vi "CreateCANWriteQueues.vi"(8 "error in (no error)":errorcluster, 10 "CAN frame":T1 {"type" items=["CAN Data", "CAN Remote"]; "identifier" format="%.0x"}, 11 "Queues":refnum<queue>) -> (0 "error out":errorcluster, 3 "Queues":refnum<queue>)   [LabVIEW 2016, in "DSI-RT.lvlib"]
uses:
  DSI-RT.lvlib
  <vilib>/RioEmbeddedCAN/RioEmbeddedCAN.llb/CANFrameControl.ctl
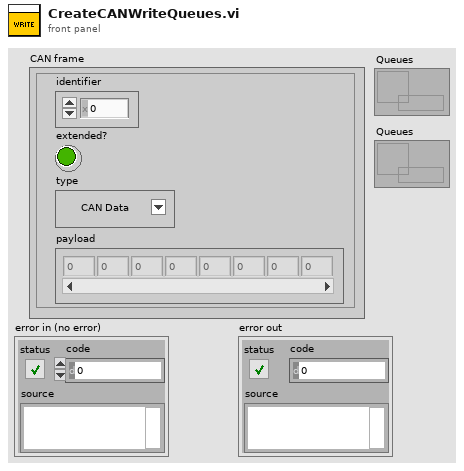
[diagram p1: front panel]
types:
  T1 = typedef "CANFrameControl.ctl" = cluster{"identifier":u32, "extended?":bool, "type":u8, "payload":u8[]}
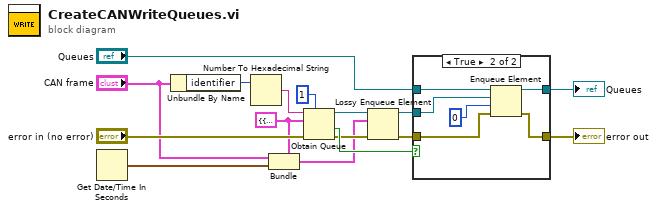
[diagram p0: block diagram]
diagram:
  w3 = cluster{"CAN frame":T1, "Timestamp":timestamp} {"CAN frame"={"identifier"=0, "extended?"=FALSE, "type"=0, "payload"=[]}, "Timestamp"=timestamp(0 s since 1904-01-01)} ("output cluster")
  n1 = Get Date/Time In Seconds() -> (seconds since 1Jan1904=w14:timestamp)
  n2 = Unbundle By Name("CAN frame") -> ("identifier"=w12:u32)
  n3 = Number To Hexadecimal String(2:w12) -> (0:w11:string)  [unwired: 1 in]
  n4 = Bundle(cluster=w3, "CAN frame"="CAN frame", "Timestamp"=w14) -> (w2:cluster{"CAN frame":T1, "Timestamp":timestamp})
  n5 = Obtain Queue(max queue size (-1, unlimited)=1, name (unnamed)=w11, element data type=w3, error in (no error)="error in (no error)") -> (queue out=w5:refnum<queue>, created new?=w9:bool, error out=w4:errorcluster)  [unwired: 1 in]
  n6 = Lossy Enqueue Element(queue=w5, element=w2, error in (no error)=w4) -> (queue out=w8:refnum<queue>, error out=w7:errorcluster)  [unwired: 2 out]
  n7 = case shown="True" w9 {
    tunnel: "Queues" -> [w17 w23]
    tunnel: w8 -> [_ w22]
    tunnel: w7 -> [w18 w21]
    tunnel: [w18 w20] -> w6
    tunnel: [w17 w19] -> w1
    frame False {
    }
    frame True {
      n8 = Enqueue Element(queue=w23, element=w22, timeout in ms (-1)=0, error in (no error)=w21) -> (queue out=w19:refnum<queue>, error out=w20:errorcluster)  [unwired: 1 out]
    }
  }
  "error out" <- w6
  "Queues" <- w1
